vi "Create Dialog.vi"(5 "Bar Visibility":T2={"Menu Bar"=FALSE, "Title Bar"=TRUE}, 6 "Calling VI Reference":refnum<vi>, 7 "Scrollbars (off)":T3, 8 "error in":errorcluster, 9 "Launch Position (Centered)":T1=enum."Centered", 10 "Dialog Behavior":T4(ring)=enum."Default", 11 "UI VI Reference (caller)":refnum<vi>) -> (0 "error out":errorcluster, 3 "Flex Dialog out":refnum<class "Flex UI Dialog.lvclass">)   [LabVIEW 2016, in "Flex UI Dialog.lvclass"]
doc: "Generates a Dialog with all the associated behavior from the input UI VI Reference.\n\nIf no reference is given, uses the calling VI."
uses:
  Flex UI Dialog.lvclass
  C:/VI Packages/Flex UI/Flex UI (Parent)/Flex UI.lvclass
  Cluster - Scrollbar Settings.ctl
  Cluster - Bar Visibility.ctl
  Enum - Launch Position.ctl
  Flex UI (Parent)/Flex UI.lvclass/Flex UI.ctl
  Flex UI Dialog.lvclass/Flex UI Dialog.ctl
  Flex UI (Parent)/Flex UI.lvclass
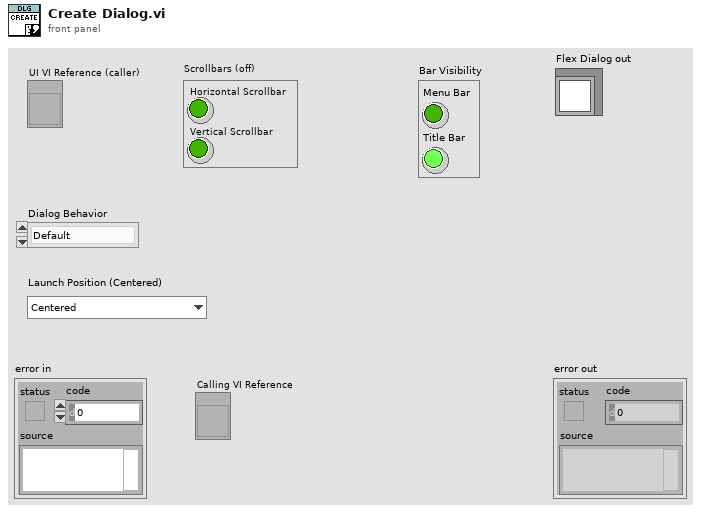
[diagram p1: front panel]
types:
  T1 = typedef "Flex UI Dialog.lvclass/Enum - Launch Position.ctl" = enum16{"Default (Last Opened)", "Centered", "Centered on Caller", "Maximized", "Hidden"}
  T2 = typedef "Flex UI Dialog.lvclass/Cluster - Bar Visibility.ctl" = cluster{"Menu Bar":bool, "Title Bar":bool}
  T3 = typedef "Flex UI Dialog.lvclass/Cluster - Scrollbar Settings.ctl" = cluster{"Horizontal Scrollbar":bool, "Vertical Scrollbar":bool}
  T4 = enum32{"Invalid", "Default", "Floating", "Floating/Auto-Hide", "Modal"}
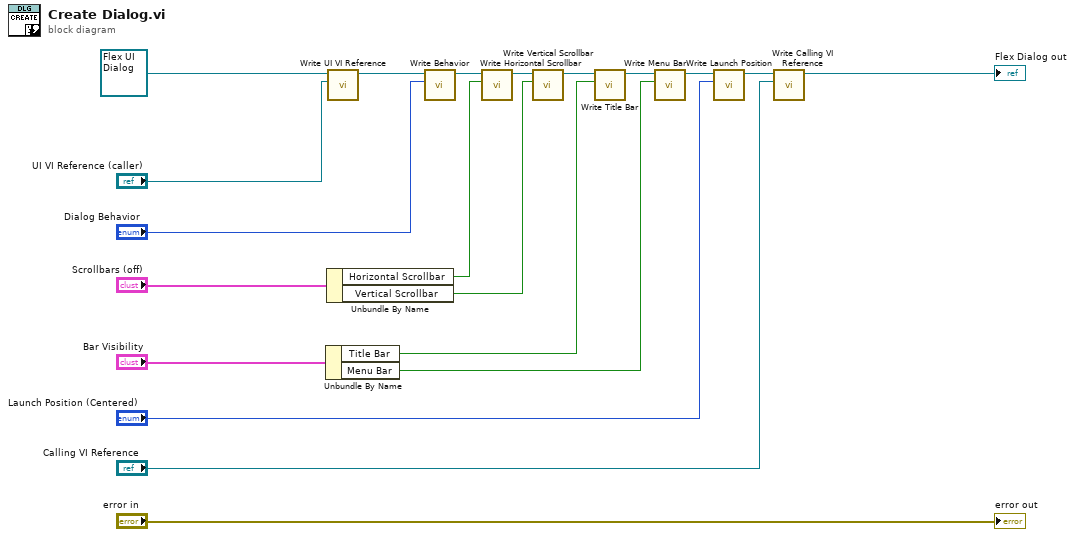
[diagram p0: block diagram]
diagram:
  n1 = Unbundle By Name("Bar Visibility") -> ("Title Bar"=w7:bool, "Menu Bar"=w6:bool)
  n2 = Unbundle By Name("Scrollbars (off)") -> ("Horizontal Scrollbar"=w10:bool, "Vertical Scrollbar"=w9:bool)
  n3 = call "Write UI VI Reference.vi"("UI VI Reference"="UI VI Reference (caller)", "Flex UI in"=refnum<class "Flex UI Dialog.lvclass"> refnum ("Flex Dialog out")) -> ("Flex UI out"=w18:refnum<class "Flex UI Dialog.lvclass">)  [unwired: 9 in]
  n4 = call "Write Behavior.vi"("Behavior"="Dialog Behavior", "Flex Dialog in"=w18) -> ("Flex Dialog out"=w12:refnum<class "Flex UI Dialog.lvclass">)  [unwired: 9 in]
  n5 = call "Write Horizontal Scrollbar.vi"("Horizontal Scrollbar"=w10, "Flex Dialog in"=w12) -> ("Flex Dialog out"=w16:refnum<class "Flex UI Dialog.lvclass">)  [unwired: 9 in]
  n6 = call "Write Vertical Scrollbar.vi"("Vertical Scrollbar"=w9, "Flex Dialog in"=w16) -> ("Flex Dialog out"=w15:refnum<class "Flex UI Dialog.lvclass">)  [unwired: 9 in]
  n7 = call "Write Title Bar.vi"("Title Bar"=w7, "Flex Dialog in"=w15) -> ("Flex Dialog out"=w14:refnum<class "Flex UI Dialog.lvclass">)  [unwired: 9 in]
  n8 = call "Write Menu Bar.vi"("Menu Bar"=w6, "Flex Dialog in"=w14) -> ("Flex Dialog out"=w13:refnum<class "Flex UI Dialog.lvclass">)  [unwired: 9 in]
  n9 = call "Write Launch Position.vi"("Launch Position"="Launch Position (Centered)", "Flex Dialog in"=w13) -> ("Flex Dialog out"=w5:refnum<class "Flex UI Dialog.lvclass">)  [unwired: 9 in]
  n10 = call "Write Calling VI Reference.vi"("Calling VI Reference"="Calling VI Reference", "Flex Dialog in"=w5) -> ("Flex Dialog out"=→"Flex Dialog out":refnum<class "Flex UI Dialog.lvclass">)  [unwired: 9 in]
  "error out" <- "error in"
